vi "Edit-advanced-param-defaults-with-dialog.vi"() -> ()   [LabVIEW 2013, in "CameraVision.lvlib" / "CV-Main.lvclass"]
uses:
  CV-Main.lvclass
  Parameters-advanced.ctl
  Configuration/Configuration-parameters-advanced.ctl
  Acquisition/Acquisition-parameters-advanced.ctl
  Correction/Correction-parameters-advanced.ctl
  Analysis/Analysis-parameters-advanced.ctl
  Temperature/Temperature-parameters-advanced.ctl
  Storage/Storage-parameters-advanced.ctl
  Storage/Storage-types-labels.ctl
  <vilib>/Utility/xml.llb/Write to XML File(string).vi
  Acquisition/CV-Acquisition.lvclass
  Analysis/CV-Analysis.lvclass
  Configuration/CV-Configuration.lvclass
  Correction/CV-Correction.lvclass
  Temperature/CV-Temperature.lvclass
  Storage/CV-Storage.lvclass
panel:
  in  "Relative save path":string="Program data\\parameters-advanced.xml"
  in  "Advanced parameters":T1={"Config params adv"={"Image border size"=1, "Framegrabber board"=0, "Framegrabber buffer"=1, "Camera config file"=path "Support files/camera-config.mcf", "Framegrabber DLL file"=path "Support files/SiSo_LabviewInterface.dll"}, "Acquis params adv"={"Image acquisition timeout factor"=1.0, "Image collection timeout factor"=2.0, "Manual trigger ID"=25, "Precision hardware counter"="Dev1/ctr0", "When to use gate signal?"=TRUE, "Minimum acquisition timeout"=1, "External timing channel"="/Dev1/PFI4", "External gating channel"="Dev1/port1/line1"}, "Correct params adv"={"2nd image mirror axis"=1, "Cross-correlation decimation"=5, "Cross-correlation algorithm"=enum."frequency domain", "Always threshold when smoothing?"=TRUE, "Threshold only 2nd camera image?"=FALSE, "Median filter type"={"Order #"=4, "Y Size"=3, "X Size"=3}, "Gaussian filter kernel size"=3, "Gaussian filter kernel number"=4}, "Analys params adv"={"Melt-pool connectivity"=FALSE, "Melt-pool characteristics"=[35, 22, 25, 0, 1, 46]}, "Temp params adv"={"Axis origin relative position"=0.5, "Regression file relative path"="Program data\\temperatureFieldRegression.dat"}, "Storage params adv"={"Storage labels"={"Original"="Original", "Corrected"="Corrected", "Binary"="Binary", "Temperature"="Temperature", "Characteristics"="Characteristics", "Mapping"="Map", "TemperatureValues"="TemperatureValues"}, "Characteristics headers"=["Average intensity [0-255]", "Peak intensity [0-255]", "Melt-pool size [mm²]", "Melt-pool aspect ratio []", "Melt-pool fragments []", "Melt-pool center X [pix]", "Melt-pool center Y [pix]", "Melt-pool orientation [cw-rad]"], "CharacteristicsTemperature headers"=["Average temperature [°C]", "Max. temperature [°C]", "Min. temperature [°C]", "Std. dev. temperature [°C]", "Data points"]}} {"Analys params adv"."Melt-pool characteristics" items=["Center of Mass X", "Center of Mass Y", "First Pixel X", "First Pixel Y", "Bounding Rect Left", "Bounding Rect Top", "Bounding Rect Right", "Bounding Rect Bottom", "Max Feret Diameter Start X", "Max Feret Diameter Start Y", "Max Feret Diameter End X", "Max Feret Diameter End Y", "Max Horiz. Segment Length Left", "Max Horiz. Segment Length Right", "Max Horiz. Segment Length Row", "-", "Bounding Rect Width", "Bounding Rect Height", "Bounding Rect Diagonal", "Perimeter", "Convex Hull Perimeter", "Holes' Perimeter", "Max Feret Diameter", "Equivalent Ellipse Major Axis", "Equivalent Ellipse Minor Axis", "Equivalent Ellipse Minor Axis (Feret)", "Equivalent Rect Long Side", "Equivalent Rect Short Side", "Equivalent Rect Diagonal", "Equivalent Rect Short Side (Feret)", "Average Horiz. Segment Length", "Average Vert. Segment Length", "Hydraulic Radius", "Waddel Disk Diameter", "-", "Area", "Holes' Area", "Particle & Holes' Area", "Convex Hull Area", "Image Area", "-", "Number of Holes", "Number of Horiz. Segments", "Number of Vert. Segments", "-", "Orientation", "Max Feret Diameter Orientation", "-", "% Area/Image Area", "% Area/(Particle & Holes' Area)", "Ratio of Equivalent Ellipse Axes", "Ratio of Equivalent Rect Sides", "-", "Elongation Factor", "Compactness Factor", "Heywood Circularity Factor", "Type Factor", "-", "Sum X", "Sum Y", "Sum XX", "Sum XY", "Sum YY", "Sum XXX", "Sum XXY", "Sum XYY", "Sum YYY", "-", "Moment of Inertia XX", "Moment of Inertia XY", "Moment of Inertia YY", "Moment of Inertia XXX", "Moment of Inertia XXY", "Moment of Inertia XYY", "Moment of Inertia YYY", "Norm. Moment of Inertia XX", "Norm. Moment of Inertia XY", "Norm. Moment of Inertia YY", "Norm. Moment of Inertia XXX", "Norm. Moment of Inertia XXY", "Norm. Moment of Inertia XYY", "Norm. Moment of Inertia YYY", "Hu Moment 1", "Hu Moment 2", "Hu Moment 3", "Hu Moment 4", "Hu Moment 5", "Hu Moment 6", "Hu Moment 7"]; "Config params adv"."Framegrabber buffer" min=1; "Config params adv"."Framegrabber board" min=0; "Config params adv"."Image border size" min=0}
  in  "Cancel":bool
  in  "OK":bool
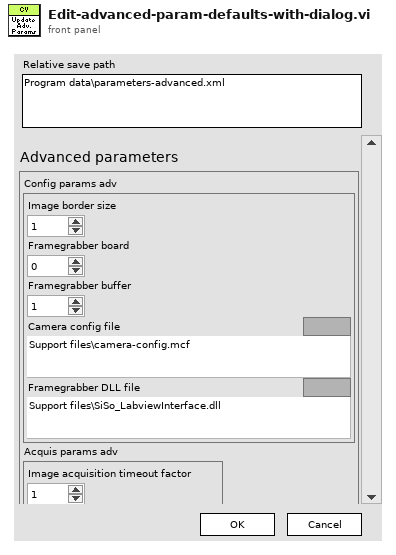
[diagram p1: front panel]
types:
  T1 = typedef "CameraVision.lvlib/CV-Main.lvclass/Parameters-advanced.ctl" = cluster{"Config params adv":T2, "Acquis params adv":T3, "Correct params adv":T4, "Analys params adv":T5, "Temp params adv":T7, "Storage params adv":T8}
  T2 = typedef "CameraVision.lvlib/CV-Configuration.lvclass/Configuration-parameters-advanced.ctl" = cluster{"Image border size":i32, "Framegrabber board":i32, "Framegrabber buffer":i32, "Camera config file":path, "Framegrabber DLL file":path}
  T3 = typedef "CameraVision.lvlib/CV-Acquisition.lvclass/Acquisition-parameters-advanced.ctl" = cluster{"Image acquisition timeout factor":dbl, "Image collection timeout factor":dbl, "Manual trigger ID":u8, "Precision hardware counter":tag, "When to use gate signal?":bool, "Minimum acquisition timeout":i32, "External timing channel":tag, "External gating channel":tag}
  T4 = typedef "CameraVision.lvlib/CV-Correction.lvclass/Correction-parameters-advanced.ctl" = cluster{"2nd image mirror axis":u32, "Cross-correlation decimation":i32, "Cross-correlation algorithm":enum32{"direct", "frequency domain"}, "Always threshold when smoothing?":bool, "Threshold only 2nd camera image?":bool, "Median filter type":cluster{"Order #":i32, "Y Size":i32, "X Size":i32}, "Gaussian filter kernel size":i32, "Gaussian filter kernel number":i32}
  T5 = typedef "CameraVision.lvlib/CV-Analysis.lvclass/Analysis-parameters-advanced.ctl" = cluster{"Melt-pool connectivity":bool, "Melt-pool characteristics":T6[]}
  T6 = typedef "Particle Parameters" = i32
  T7 = typedef "CameraVision.lvlib/CV-Temperature.lvclass/Temperature-parameters-advanced.ctl" = cluster{"Axis origin relative position":dbl, "Regression file relative path":string}
  T8 = typedef "CameraVision.lvlib/CV-Storage.lvclass/Storage-parameters-advanced.ctl" = cluster{"Storage labels":T9, "Characteristics headers":string[], "CharacteristicsTemperature headers":string[]}
  T9 = typedef "CameraVision.lvlib/CV-Storage.lvclass/Storage-types-labels.ctl" = cluster{"Original":string, "Corrected":string, "Binary":string, "Temperature":string, "Characteristics":string, "Mapping":string, "TemperatureValues":string}
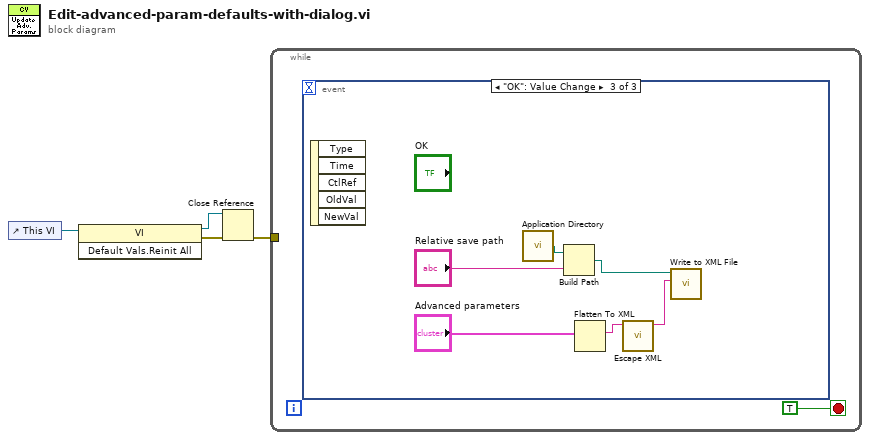
[diagram p0: block diagram]
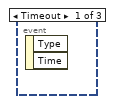
[diagram p2: hidden frame]
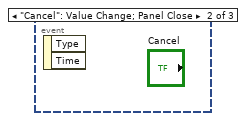
[diagram p3: hidden frame]
diagram:
  n1 = control-ref of="This VI"() -> (w4:refnum<vi>)
  n2 = invoke class="VI" method="Default Vals.Reinit All"(reference=w4) -> (reference out=w1:refnum<vi>, error out=w3:errorcluster)  [unwired: 2 in, 1 out]
  n3 = Close Reference(reference=w1, error in (no error)=w3) -> (error out=w2:errorcluster)
  n4 = while {
    tunnel: w2 -> [_]
    stop <- TRUE stop-if-true
    n5 = event shown="[2] \"OK\": Value Change" {
      selector: _ -> [_ _ _]
      dyn-events: _ -> [_ _ _]
      timeout: _ -> [_ _ _]
      event Timeout {
        n6 = event-data() -> ()  [unwired: 1 in, 2 out]
      }
      event "Cancel": Value Change; Panel Close {
        n7 = event-data() -> ()  [unwired: 1 in, 2 out]
      }
      event "OK": Value Change {
        n8 = event-data() -> ()  [unwired: 1 in, 5 out]
        n9 = call <vilib>:"Application Directory.vi"() -> ("Application Directory"=w8:path)
        n10 = Build Path(base path=w8, name or relative path="Relative save path") -> (appended path=w10:path)
        n11 = Flatten To XML(anything="Advanced parameters") -> (xml string=w9:string)
        n12 = call <vilib>:"Escape XML.vi"("XML String In"=w9) -> ("XML String Out"=w11:string)  [unwired: 9 in, 1 out]
        n13 = call-poly <vilib>:"Write to XML File.vi"("XML Input"=w11, "XML File Path"=w10) -> ()  [unwired: 7 in, 3 out]
      }
    }
  }
